vi "Q*.vi"(1 "quaternion":T1) -> (0 "quaternion*":T1)   [LabVIEW 2024]
uses:
  <vilib>/robotics/Kinematics/Quaternion.ctl
  <vilib>/robotics/Kinematics/NI_Kinematics.lvlib
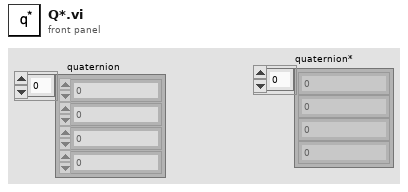
[diagram p1: front panel]
types:
  T1 = typedef "NI_Kinematics.lvlib/Quaternion.ctl" = dbl[]
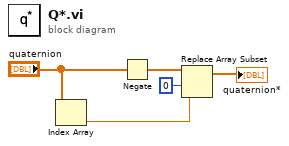
[diagram p0: block diagram]
diagram:
  n1 = Index Array(array="quaternion") -> (element=w2:dbl)  [unwired: 1 in]
  n2 = Negate(x="quaternion") -> (-x=w4:T1)
  n3 = Replace Array Subset(array=w4, new element=w2, index=0) -> (→"quaternion*":T1)
